vi "test VerifyByValue.vi"(8 "error in (no error)":errorcluster, 11 "TestCase in":refnum<class "Test Numeric Test Object.lvclass">) -> (0 "error out":errorcluster, 3 "TestCase out":refnum<class "Test Numeric Test Object.lvclass">)   [LabVIEW 2009, in "Test Numeric Test Object.lvclass"]
uses:
  Test Numeric Test Object.lvclass
  Test Numeric Test Object.lvclass/Test Numeric Test Object.ctl
  Numeric Test Object/Numeric Test Object.lvclass
  <vilib>/addons/_JKI Toolkits/VI Tester/TestCase.llb/TestCase.lvclass
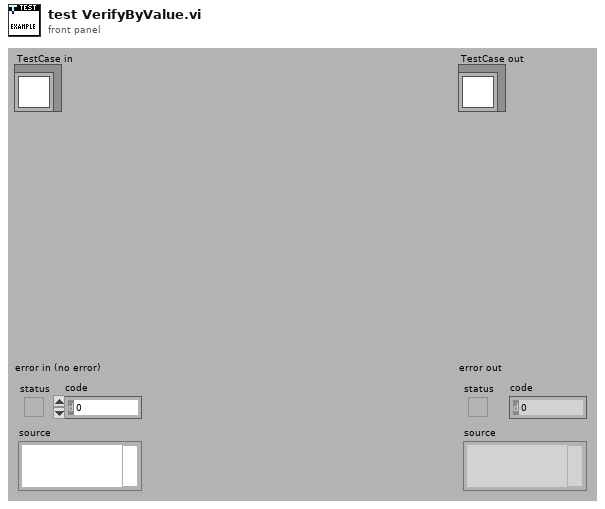
[diagram p1: front panel]
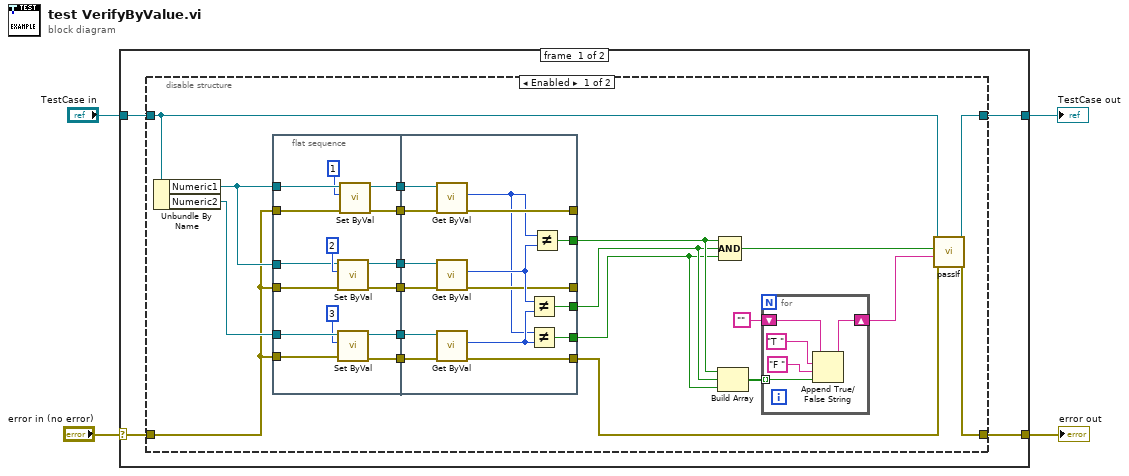
[diagram p0: block diagram]
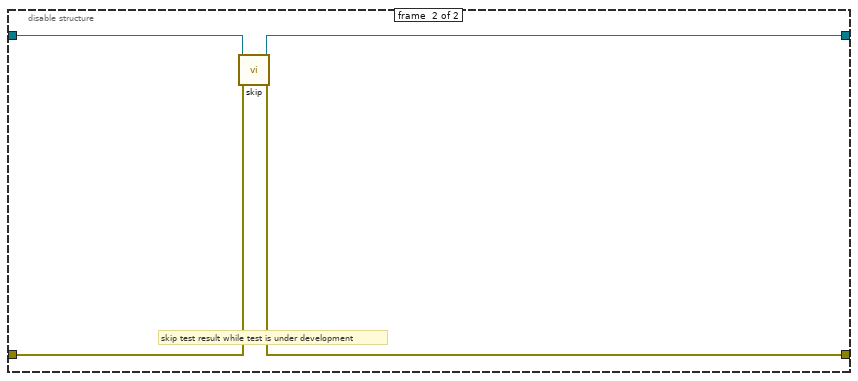
[diagram p2: hidden frame]
diagram:
  n1 = case shown="No Error" "error in (no error)" {
    selector: "error in (no error)" -> [w6 w69]
    tunnel: [w5 w69] -> w3
    tunnel: [w7 w68] -> w1
    tunnel: "TestCase in" -> [w8 w68]
    frame #0 {
      n2 = disable-structure shown="Enabled" {
        disable-tunnel: w8 -> [w26 w67]
        disable-tunnel: [w28 w64] -> w7
        disable-tunnel: w6 -> [w19 w66]
        disable-tunnel: [w27 w65] -> w5
        frame #0 {
          n3 = Unbundle By Name(w26) -> ("Numeric1"=w20:refnum<class "Numeric Test Object.lvclass">, "Numeric2"=w25:refnum<class "Numeric Test Object.lvclass">)
          n4 = flat-sequence {
            tunnel: w25 -> [w42]
            tunnel: w20 -> [w39]
            tunnel: w19 -> [w37]
            tunnel: w20 -> [w35]
            tunnel: w19 -> [w34]
            tunnel: w19 -> [w33]
            tunnel: [w43] -> w18
            tunnel: [w41] -> w17
            tunnel: [w32] -> w16
            tunnel: [w31] -> w15
            tunnel: [w30] -> w14
            tunnel: [w29] -> w13
            tunnel: w18 -> [w58]
            tunnel: w17 -> [w57]
            tunnel: w16 -> [w56]
            tunnel: w15 -> [w55]
            tunnel: w14 -> [w54]
            tunnel: w13 -> [w53]
            tunnel: [w51] -> _
            tunnel: [w50] -> _
            tunnel: [w49] -> w11
            tunnel: [w48] -> w10
            tunnel: [w47] -> w12
            tunnel: [w44] -> w9
            frame #0 {
              n5 = call-dynamic "Set ByVal.vi"("error in (no error)"=w34, "Int"=2, "Numeric in"=w35) -> ("error out"=w31:errorcluster, "Numeric out"=w32:refnum<class "Numeric Test Object.lvclass">)  [unwired: 7 in]
              n6 = call-dynamic "Set ByVal.vi"("error in (no error)"=w37, "Int"=3, "Numeric in"=w42) -> ("error out"=w29:errorcluster, "Numeric out"=w30:refnum<class "Numeric Test Object.lvclass">)  [unwired: 7 in]
              n7 = call-dynamic "Set ByVal.vi"("error in (no error)"=w33, "Int"=1, "Numeric in"=w39) -> ("error out"=w41:errorcluster, "Numeric out"=w43:refnum<class "Numeric Test Object.lvclass">)  [unwired: 7 in]
            }
            frame #1 {
              n8 = call-dynamic "Get ByVal.vi"("error in (no error)"=w57, "Numeric in"=w58) -> ("error out"=w51:errorcluster, "Int"=w45:i32)  [unwired: 7 in, 1 out]
              n9 = call-dynamic "Get ByVal.vi"("error in (no error)"=w55, "Numeric in"=w56) -> ("error out"=w50:errorcluster, "Int"=w52:i32)  [unwired: 7 in, 1 out]
              n10 = call-dynamic "Get ByVal.vi"("error in (no error)"=w53, "Numeric in"=w54) -> ("error out"=w49:errorcluster, "Int"=w46:i32)  [unwired: 7 in, 1 out]
              n11 = Not Equal?(x=w52, y=w46) -> (x != y?=w48:bool)
              n12 = Not Equal?(x=w45, y=w46) -> (x != y?=w44:bool)
              n13 = Not Equal?(x=w45, y=w52) -> (x != y?=w47:bool)
            }
          }
          n14 = Build Array(w12, w10, w9) -> (w23:bool[])
          n15 = Compound Arithmetic op=AND(w12, w10, w9) -> (w24:bool)
          n16 = for {
            tunnel: w23 -> [w63] mode=indexing
            shift-right: [w62] -> w21
            shift-left: "" -> [w59]
            n17 = Append True/False String(1:w63, 2:"F " ("false string"), 3:"T " ("true string"), 4:w59) -> (0:w62:string)
          }
          n18 = call-dynamic "passIf.vi"("error in (no error)"=w11, "message (\"\")"=w21, "pass"=w24, "TestCase in"=w26) -> ("error out"=w27:errorcluster, "TestCase out"=w28:refnum<class "Test Numeric Test Object.lvclass">)  [unwired: 6 in]
        }
        frame #1 {
          # "skip test result while test is under development"
          n19 = call <vilib>:"skip.vi"("error in (no error)"=w66, "TestCase in"=w67) -> ("error out"=w65:errorcluster, "TestCase out"=w64:refnum<class "Test Numeric Test Object.lvclass">)  [unwired: 8 in]
        }
      }
    }
    frame #1 {
    }
  }
  "error out" <- w3
  "TestCase out" <- w1
